vi "measresult save.vi"(8 "error in (no error)":errorcluster, 10 "sort index":i32, 11 "measresult":T1 {"measdata"."Current Magnetic\nField\n(430 TCP reading)"."phi (deg)" format="%#_3g"}) -> (0 "error out":errorcluster)   [LabVIEW 2013]
uses:
  measresult cluster.ctl
  measconfig cluster.ctl
  measurement sweep parameter.ctl
  devices/magnet/magnet polar field.ctl
  measdata cluster.ctl
  devices/magnet/AMI reading polar field.ctl
  devices/vna/vna s-parameters.ctl
  <vilib>/Utility/VariantDataType/VariantType.lvlib
panel:
  # "List of measurement data for the S-parameters."
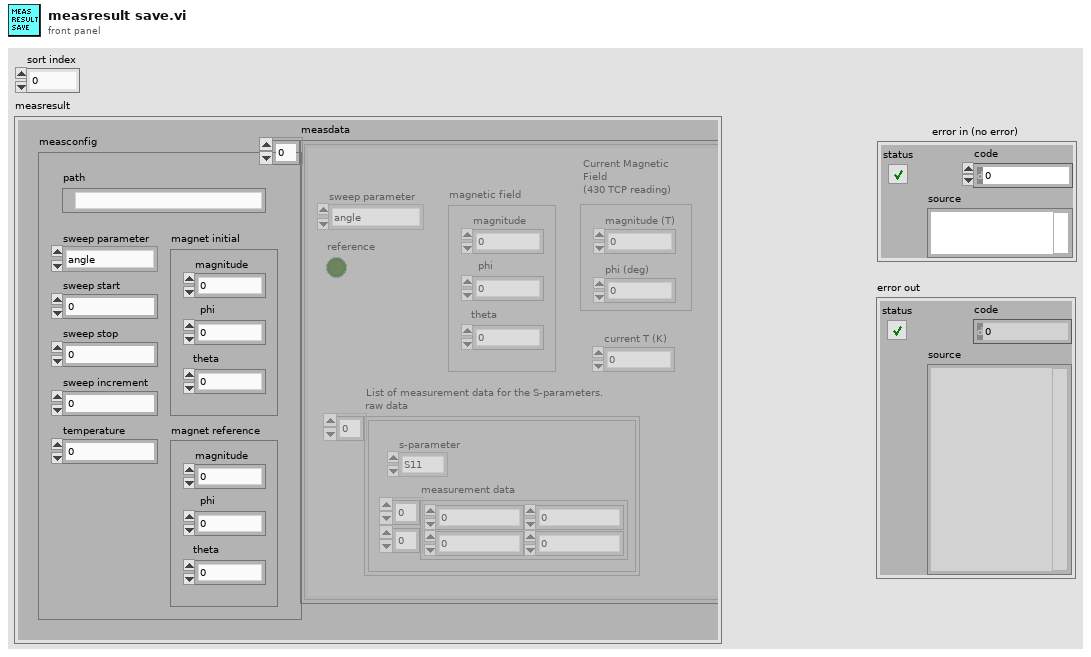
[diagram p1: front panel]
types:
  T1 = typedef "measresult cluster.ctl" = cluster{"measconfig":T2, "measdata":T5[]}
  T2 = typedef "measconfig cluster.ctl" = cluster{"sweep parameter":T3, "sweep start":dbl, "sweep stop":dbl, "sweep increment":dbl, "temperature":dbl, "path":path, "magnet initial":T4, "magnet reference":T4}
  T3 = typedef "measurement sweep parameter.ctl" = enum16{"angle", "magnetic field"}
  T4 = typedef "magnet polar field.ctl" = cluster{"magnitude":dbl, "phi":dbl, "theta":dbl}
  T5 = typedef "measdata cluster.ctl" = cluster{"raw data":cluster{"measurement data":dbl[][], "s-parameter":enum16{"S11", "S12", "S21", "S22"}}[], "magnetic field":T4, "reference":bool, "sweep parameter":T3, "Current Magnetic\nField\n(430 TCP reading)":T6, "current T (K)":dbl}
  T6 = typedef "AMI reading polar field.ctl" = cluster{"magnitude (T)":dbl, "phi (deg)":dbl}
  T7 = enum16{"open", "replace", "create", "open or create", "replace or create", "replace or create with confirmation"}
  T8 = typedef "vna s-parameters.ctl" = enum16{"S11", "S12", "S21", "S22"}
  T9 = cluster{"measurement data":dbl[][], "s-parameter":enum16{"S11", "S12", "S21", "S22"}}[]
  T10 = cluster{"measurement data":dbl[][], "s-parameter":enum16{"S11", "S12", "S21", "S22"}}
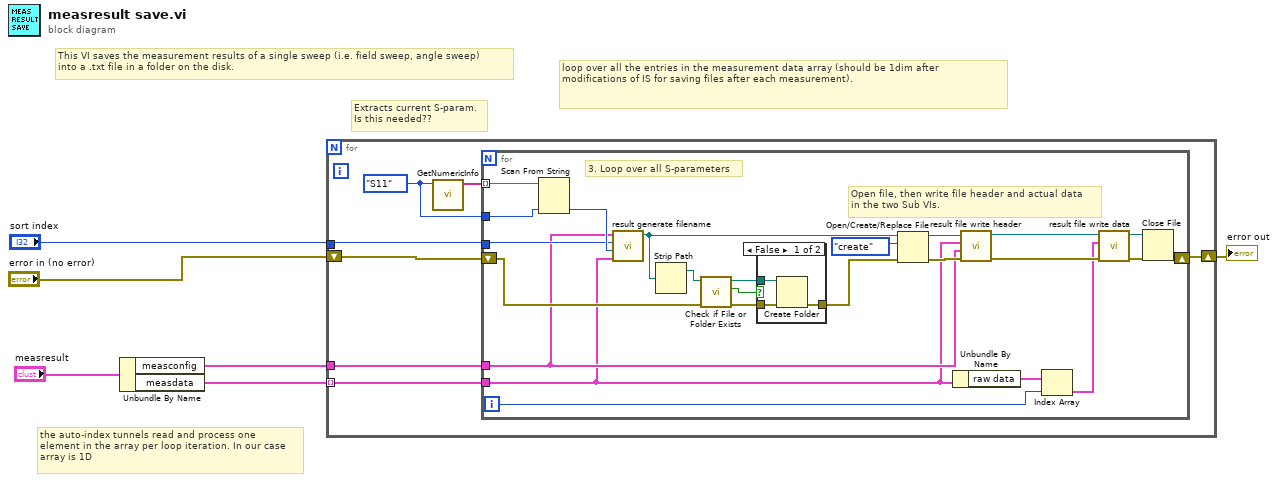
[diagram p0: block diagram]
diagram:
  # "the auto-index tunnels read and process one \nelement in the array per loop iteration. In our case\narray is 1D"
  # "Extracts current S-param.\nIs this needed??"
  # "loop over all the entries in the measurement data array (should be 1dim after modifications of IS for saving files after each measurement)."
  # "This VI saves the measurement results of a single sweep (i.e. field sweep, angle sweep) \ninto a .txt file in a folder on the disk."
  n1 = Unbundle By Name("measresult") -> ("measconfig"=w4:T2, "measdata"=w5:T5[])
  n2 = for {
    shift-right: [w8] -> w3
    shift-left: "error in (no error)" -> [w9]
    tunnel: w5 -> [w10] mode=indexing
    tunnel: w4 -> [w11]
    tunnel: "sort index" -> [w7]
    w12 = vna_s-parameters."S11" ("vna s-parameters")
    n3 = call <vilib>:"GetNumericInfo.vi"("Variant"=w12) -> ("EnumNames"=w13:string[])  [unwired: 7 in, 3 out]
    n4 = for {
      tunnel: w13 -> [w37] mode=indexing
      tunnel: w12 -> [w36]
      tunnel: w11 -> [w18]
      tunnel: w10 -> [w17]
      shift-right: [w29] -> w8
      shift-left: w9 -> [w26]
      tunnel: w7 -> [w19]
      i -> [w15]
      # "3. Loop over all S-parameters"
      # "Open file, then write file header and actual data\nin the two Sub VIs."
      n5 = Scan From String(input string=w37, default 1=w36) -> (output 1=w20:T8)  [unwired: 3 in, 3 out]
      n6 = call "result generate filename.vi"("measdata definition"=w17, "vna s-parameters"=w20, "sort index"=w19, "measurement definition"=w18) -> ("result path"=w28:path)  [unwired: 7 in]
      n7 = Strip Path(path=w28) -> (stripped path=w27:path)  [unwired: 1 out]
      n8 = call <vilib>:"Check if File or Folder Exists.vi"("error in (no error)"=w26, "path"=w27) -> ("error out"=w24:errorcluster, "file or folder exists?"=w23:bool, "dup path"=w25:path)  [unwired: 7 in]
      n9 = case shown="False" w23 {
        tunnel: w25 -> [w40 _]
        tunnel: w24 -> [w39 w41]
        tunnel: [w38 w41] -> w22
        frame False {
          n10 = Create Folder(path (use dialog)=w40, error in=w39) -> (error out=w38:errorcluster)  [unwired: 1 in, 2 out]
        }
        frame True {
        }
      }
      n11 = Open/Create/Replace File(file path (use dialog)=w28, error in=w22, operation (0:open)=T7."create") -> (refnum out=w35:refnum<file>, error out=w34:errorcluster)  [unwired: 3 in, 1 out]
      n12 = Unbundle By Name(w17) -> ("raw data"=w16:T9)
      n13 = call "result file write header.vi"("error in (no error)"=w34, "measurement definition"=w18, "measdata definition"=w17, "refnum"=w35) -> ("error out"=w33:errorcluster, "refnum out"=w32:refnum<file>)  [unwired: 6 in]
      n14 = Index Array(array=w16, index=w15) -> (element=w14:T10)
      n15 = call "result file write data.vi"("error in (no error)"=w33, "raw data"=w14, "refnum"=w32) -> ("error out"=w30:errorcluster, "refnum out"=w31:refnum<file>)  [unwired: 7 in]
      n16 = Close File(refnum=w31, error in=w30) -> (error out=w29:errorcluster)  [unwired: 1 out]
    }
  }
  "error out" <- w3
